vi "daq2.vi"() -> ()   [LabVIEW 2011]
panel:
  in  "stop":bool
  out "ledn3":bool
  out "ledn2":bool
  out "ledn1":bool
  in  "Led 3":bool
  in  "Led 2":bool
  in  "Led 1":bool
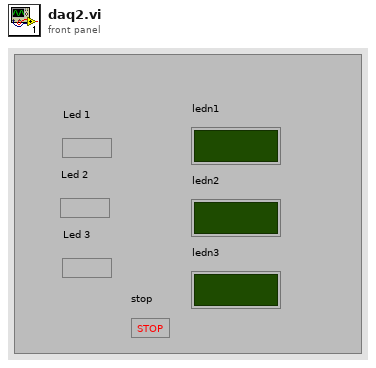
[diagram p1: front panel]
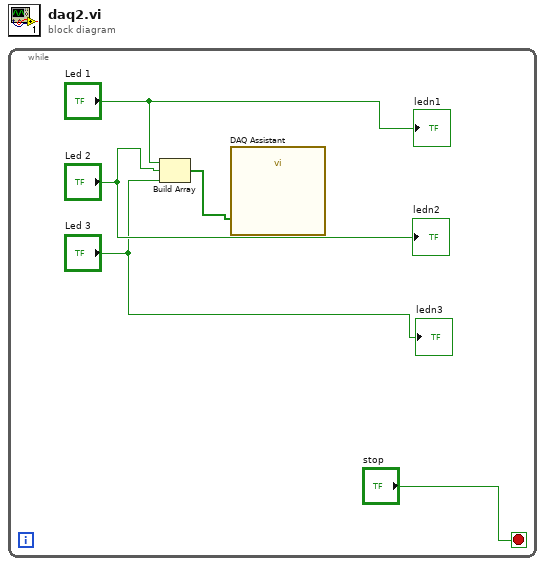
[diagram p0: block diagram]
diagram:
  n1 = while {
    stop <- "stop" stop-if-true
    n2 = Build Array "Build Array"("Led 1", "Led 2", "Led 3") -> (w1:bool[])
    n3 = call "DAQ Assistant"("data"=w1) -> ()  [unwired: 17 in, 2 out]
    "ledn1" <- "Led 1"
    "ledn2" <- "Led 2"
    "ledn3" <- "Led 3"
  }
